vi "getDigitalOutputsStatus.vi"(0 "Controller in":refnum<class "_Controller.lvclass">, 2 "do (single)":T2, 4 "get_all? (def=F)":bool, 5 "error in (no error)":errorcluster) -> (14 "Controller out":refnum<class "_Controller.lvclass">, 15 "dig_val (single only)":bool, 16 "do_items":T1[](array[typedef]), 17 "raw_do_value":string, 19 "error out":errorcluster)   [LabVIEW 2020, in "classes.lvlib" / "_Controller.lvclass"]
doc: "Retrieves the status of a digital output channel (or retrieves the status of all DO channels if \"get_all?\" is set to TRUE.\n\nProduced By:\n\n<B>Kod Integrations, LLC</B>\n4835 Marianne Drive\nMount Airy, MD 21771\nhttp://www.kodintegrations.com\nemail: info@kodintegrations.com\nphone: (240) 687-1288"
uses:
  _Controller.lvclass
  digital_output.ctl
  digital_output_item.ctl
  commands.ctl
  common.lvlib
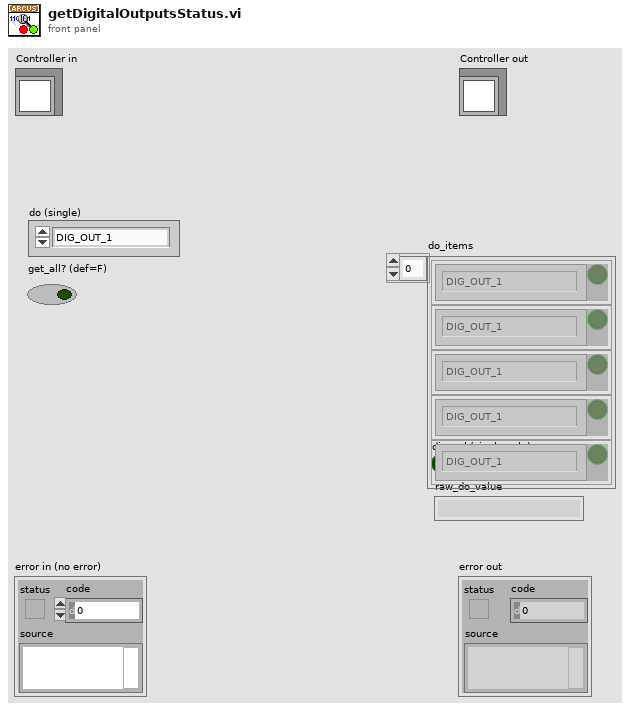
[diagram p1: front panel]
types:
  T1 = typedef "common.lvlib/digital_output_item.ctl" = cluster{"item":T2, "status":bool}
  T2 = typedef "common.lvlib/digital_output.ctl" = enum16{"DIG_OUT_1", "DIG_OUT_2", "DIG_OUT_3", "DIG_OUT_4", "DIG_OUT_5", "DIG_OUT_6", "DIG_OUT_7", "DIG_OUT_8"}
  T3 = typedef "common.lvlib/commands.ctl" = enum16{"clear error", "constant jog(-)", "constant jog(+)", "get acceleration", "get actual current", "get device name", "get digital input status", "get digital inputs status", "get digital output status", "get digital outputs status", "get firmware ver", "get high speed", "get idle current", "get low speed", "get micro step", "get motor status", "get move mode", "get polarity", "get position", "get product id", "get power status", "get run current", "get status", "home(-)", "home(+)", "move to position", "power down", "power up", "set acceleration", "set device id", "set digital output", "set digital outputs", "set high speed", "set idle current", "set low speed", "set move mode absolute", "set move mode increment", "set polarity", "set position", "set run current", "stop immediate", "stop slow", "store to memory"}
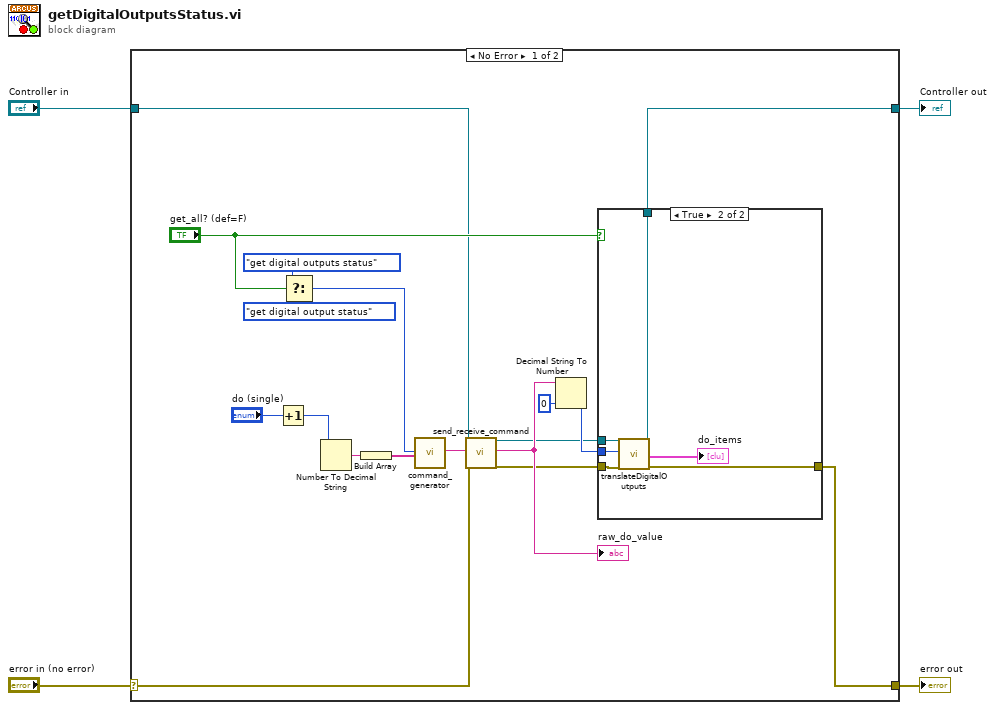
[diagram p0: block diagram]
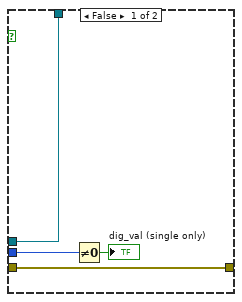
[diagram p2: hidden frame]
diagram:
  n1 = case shown="No Error" "error in (no error)" {
    selector: "error in (no error)" -> [w7 w34]
    tunnel: [w6 w34] -> w3
    tunnel: [w12 w33] -> w1
    tunnel: "Controller in" -> [w13 w33]
    frame No Error {
      n2 = Increment(x="do (single)") -> (x+1=w14:T2)
      n3 = Select(t=commands."get digital outputs status" ("command"), s="get_all? (def=F)", f=commands."get digital output status" ("command")) -> (s? t:f=w11:T3)
      n4 = Number To Decimal String(number=w14) -> (decimal integer string=w15:string)  [unwired: 1 in]
      n5 = Build Array(w15) -> (w10:string[])
      n6 = call "command_generator.vi"("cmd (in)"=w11, "params (in)"=w10) -> ("ASCII_cmd (out)"=w9:string)  [unwired: 17 in]
      n7 = call "send_receive_command.vi"("reference (in)"=w13, "ASCII Command (in)"=w9, "error in (no error)"=w7) -> ("reference (out)"=w5:refnum<class "_Controller.lvclass">, "response (out)"=w22:string, "error out"=w8:errorcluster)  [unwired: 12 in, 2 out]
      "raw_do_value" <- w22
      n8 = Decimal String To Number(string=w22, default (0L)=u32 0 ("default (0 I32)")) -> (number=w18:u32)  [unwired: 1 in, 1 out]
      n9 = case shown="True" "get_all? (def=F)" {
        tunnel: w18 -> [w26 w32]
        tunnel: [w24 w30] -> w12
        tunnel: w8 -> [w23 w29]
        tunnel: [w23 w28] -> w6
        tunnel: w5 -> [w24 w27]
        frame False {
          n10 = Not Equal To 0?(x=w26) -> (x != 0?=→"dig_val (single only)":bool)
        }
        frame True {
          n11 = call-dynamic "translateDigitalOutputs.vi"("Controller in"=w27, "DO_value (in)"=w32, "error in (no error)"=w29) -> ("Controller out"=w30:refnum<class "_Controller.lvclass">, "DO_items (out)"=→"do_items":T1[], "error out"=w28:errorcluster)  [unwired: 13 in, 1 out]
        }
      }
    }
    frame Error {
    }
  }
  "error out" <- w3
  "Controller out" <- w1
